vi "write int32.vi"() -> ()   [LabVIEW 2019]
uses:
  <vilib>/RTI DDS Toolkit/Types/RTI DDS Advanced Writer Configuration.ctl
  <vilib>/RTI DDS Toolkit/VIs/AdvancedCreateWriter_NumI32.vi
  <vilib>/RTI DDS Toolkit/VIs/Write_NumI32.vi
  <vilib>/RTI DDS Toolkit/Library/LVDDS_library.lvlib
panel:
  in  "Advanced Writer Configuration":T1={"typeName"="std_msgs::msg::dds_::Int32_", "keyName"="", "domainParticipantQoSProfile"="", "dataWriterQoSProfile"="", "forceArrayMapping?"=FALSE, "forceUnboundedString?"=FALSE}
  in  "stop":bool
  in  "Dial":u32(knob)=961 scale=0.0..1000.0
  out "Waveform Chart":i32(graph)=16
  in  "Topic Name":string="rt/labviewint"
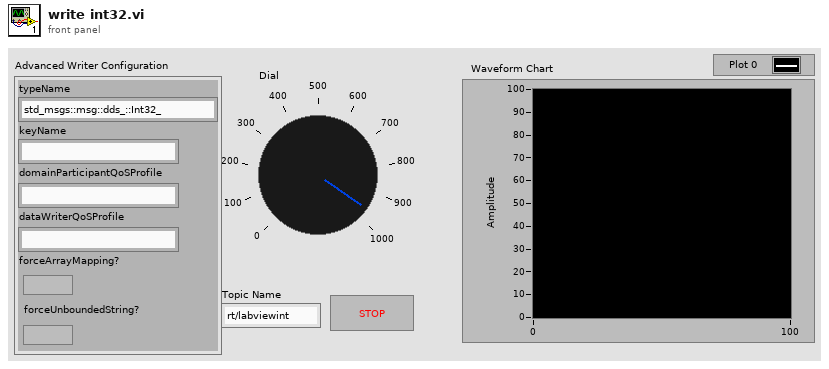
[diagram p1: front panel]
types:
  T1 = typedef "LVDDS_library.lvlib/RTI DDS Advanced Writer Configuration.ctl" = cluster{"typeName":string, "keyName":string, "domainParticipantQoSProfile":string, "dataWriterQoSProfile":string, "forceArrayMapping?":bool, "forceUnboundedString?":bool}
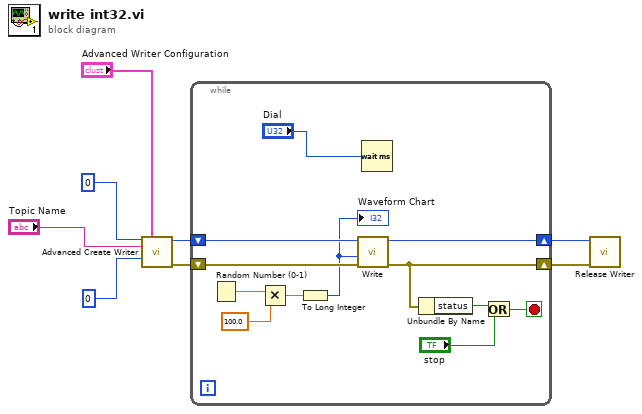
[diagram p0: block diagram]
diagram:
  n1 = call-poly <vilib>:"Advanced Create Writer.vi"("Domain Id"=u32 0, "Advanced Writer Configuration"="Advanced Writer Configuration", "Topic Name"="Topic Name", "Data Type"=0) -> ("DDS Object Ref"=w5:u64, "error out"=w8:errorcluster)  [unwired: 10 in]
  n2 = while {
    shift-right: [w17] -> w7
    shift-left: w8 -> [w20]
    shift-right: [w19] -> w6
    shift-left: w5 -> [w18]
    stop <- w14 stop-if-true
    n3 = Random Number (0-1)() -> (number: 0 to 1=w11:dbl)
    n4 = Multiply(x=w11, y=100.0) -> (x*y=w9:dbl)
    n5 = To Long Integer(number=w9) -> (32bit integer=w12:i32)
    "Waveform Chart" <- w12
    n6 = call-poly <vilib>:"Write.vi"("error in (no error)"=w20, "Data"=w12, "DDS Object Ref in"=w18) -> ("error out"=w17:errorcluster, "DDS Object Ref out"=w19:u64)  [unwired: 7 in]
    n7 = Wait (ms)(milliseconds to wait="Dial") -> ()  [unwired: 1 out]
    n8 = Unbundle By Name(w17) -> ("status"=w15:bool)
    n9 = Or(x=w15, y="stop") -> (x .or. y?=w14:bool)
  }
  n10 = call <vilib>:"Release Writer.vi"("error in (no error)"=w7, "DDS Object Ref"=w6) -> ()  [unwired: 9 in, 1 out]
